vi "ReadValByRefNamedU16.vi"(0 "Control Ref":refnum<vi>, 2 "Type In":u16, 11 "error in":errorcluster caption="entrée d'erreur") -> (4 "Chaînes []":string[](array[string]), 6 "Valeur":u16, 8 "StringAtIdx":string, 15 "error out":errorcluster caption="sortie d'erreur")   [LabVIEW 2019]
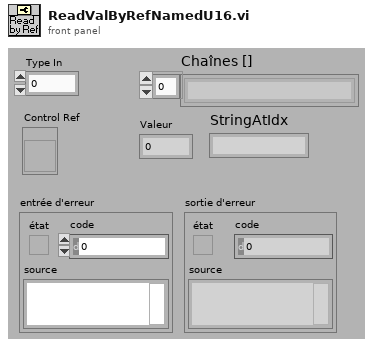
[diagram p1: front panel]
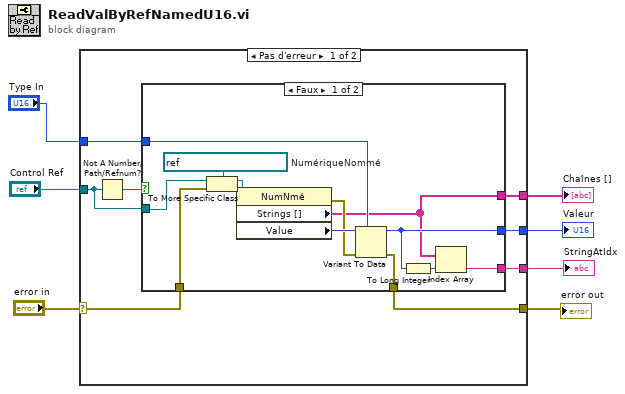
[diagram p0: block diagram]
diagram:
  n1 = case shown="Pas d'erreur" "error in" {
    selector: "error in" -> [w12 w31]
    tunnel: "Control Ref" -> [w14 _]
    tunnel: [w13 _] -> w6
    tunnel: [w11 w31] -> w4
    tunnel: "Type In" -> [w10 _]
    tunnel: [w9 _] -> w2
    tunnel: [w8 _] -> w1
    frame No Error {
      n2 = Not A Number/Path/Refnum?(number/path/refnum=w14) -> (NaN/Path/Refnum?=w15:bool)
      n3 = case shown="Faux" w15 {
        tunnel: w14 -> [w20 _]
        tunnel: [w19 w29] -> w13
        tunnel: w12 -> [w21 w30]
        tunnel: [w28 w30] -> w11
        tunnel: w10 -> [w27 w29]
        tunnel: [w16 _] -> w9
        tunnel: [w18 _] -> w8
        frame False {
          w24 = refnum<vi> refnum  # NumériqueNommé
          n4 = To More Specific Class(target class=w24, reference=w20, error in=w21) -> (specific class reference=w25:refnum<vi>, error out=w26:errorcluster)
          n5 = property class="NumNmé"(reference=w25, error in=w26) -> (error out=w22:errorcluster, "Strings []"=w16:string[], "Value"=w23:variant)  [unwired: 1 out]
          n6 = Variant To Data(error in=w22, type=w27, Variant=w23) -> (data=w19:u16, error out=w28:errorcluster)
          n7 = To Long Integer(number=w19) -> (32bit integer=w17:i32)
          n8 = Index Array(array=w16, index=w17) -> (element=w18:string)
        }
        frame True {
        }
      }
    }
    frame Error {
    }
  }
  "Valeur" <- w6
  "error out" <- w4
  "Chaînes []" <- w2
  "StringAtIdx" <- w1
